vi "LVClass_Camera get size.vi"(0 "Camera in":refnum<class "Camera.lvclass">, 11 "error in (no error)":errorcluster) -> (4 "Camera out":refnum<class "Camera.lvclass">, 6 "size":T2, 8 "Number of bits":T1, 15 "error out":errorcluster)   [LabVIEW 2020, in "Camera.lvclass"]
doc: "Get Camera dimensions and depth.\n\n<B>CameraIn</B> : Camera object.\n<B>CameraOut</B> : Camera object.\n<B>size</B> : Camera size (width, height).\n<B>bit_depth</B> : Camera bits depth."
uses:
  Camera.lvclass
  Controls/Point2D.ctl
  Controls/Data alignment enum.ctl
  Camera.lvclass/Camera.ctl
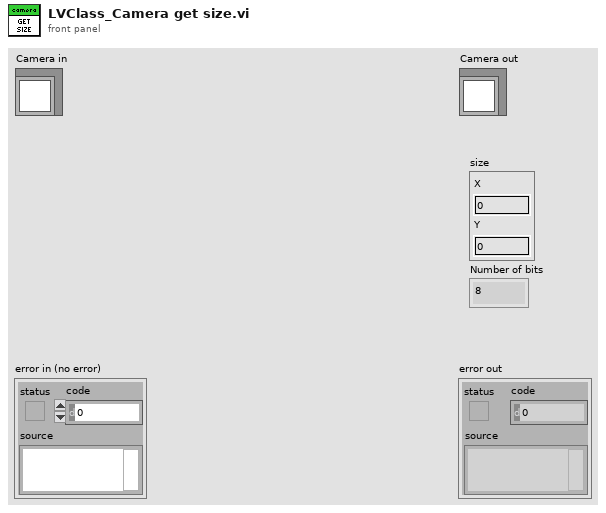
[diagram p1: front panel]
types:
  T1 = typedef "Data alignment enum.ctl" = enum16{"8", "16", "32"}
  T2 = typedef "Point2D.ctl" = cluster{"X":u32, "Y":u32}
  T3 = typedef "ClassID.ctl" = i64
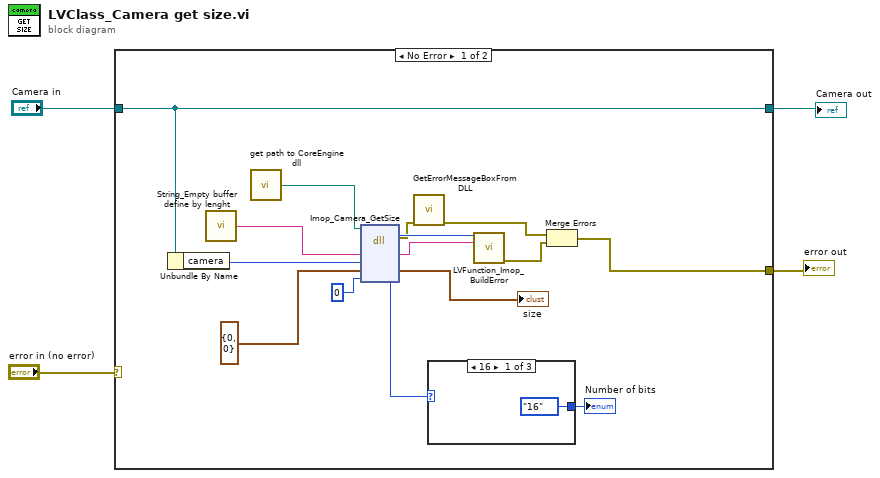
[diagram p0: block diagram]
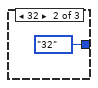
[diagram p2: hidden frame]
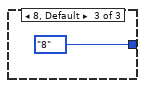
[diagram p3: hidden frame]
diagram:
  n1 = case shown="No Error" "error in (no error)" {
    selector: "error in (no error)" -> [_ w24]
    tunnel: [w9 w24] -> w1
    tunnel: [w5 w23] -> w2
    tunnel: "Camera in" -> [w5 w23]
    frame No Error {
      n2 = Unbundle By Name(w5) -> ("camera"=w16:T3)
      n3 = call "String_Empty buffer define by lenght.vi"() -> ("Empty buffer"=w19:string)  [unwired: 1 in]
      n4 = call "get path to CoreEngine dll.vi"() -> ("path to wavekit library"=w15:path)  [unwired: 14 in, 1 out]
      n5 = dll-call lib="D:/soft/HASO_v3/SVN_trunk/ImOpCoreEngine4_LV2011/DLLs/c_interface_vc100.dll" fn="Imop_Camera_GetSize"(path in=w15, "message"=w19, "Camera"=w16, "size"=T2 {"X"=0, "Y"=0} ("image_size"), "nb_bits"=u16 0) -> (error out=w13:errorcluster, "return type"=w18:i32, "message"=w17:string, "size"=→"size":T2, "nb_bits"=w12:u16)  [unwired: 3 in, 1 out]
      n6 = call "GetErrorMessageBoxFromDLL.vi"("error IN"=w13) -> ("error OUT"=w11:errorcluster)  [unwired: 10 in]
      n7 = case shown="16" w12 {
        tunnel: [Data_alignment_enum."16" ("Number of bits") Data_alignment_enum."32" ("Number of bits") Data_alignment_enum."8" ("Number of bits")] -> w6
        frame 16 {
        }
        frame 32 {
        }
        frame 8, Default {
        }
      }
      "Number of bits" <- w6
      n8 = call "LVFunction_Imop_BuildError.vi"("code"=w18, "String to Prepend to source (\"\")"=w17) -> ("error out"=w10:errorcluster)  [unwired: 13 in]
      n9 = Merge Errors(w11, w10) -> (w9:errorcluster)
    }
    frame Error {
    }
  }
  "error out" <- w1
  "Camera out" <- w2
